vi "Temperature_Analysis.vi"(0 "Temperature_Thresholds":T3, 5 "Boolean":bool) -> (8 "Analysis_Graph":dbl[](graph), 10 "Temperature_Chart":dbl(graph), 15 "Analysis_Data":T2)   [LabVIEW 2020]
doc: "This Vi will act as a temperature analysis VI in which there will be random generation of temperature and then temperature is analysed based on the user inputted threshold input and indicated to the users"
uses:
  Typedefs/Temperature Thresholds.ctl
  Typedefs/AnalysedOutputData.ctl
  Typedefs/Alert_Indicators.ctl
  <vilib>/numeric/Random Number (Range) DBL.vi
panel:
  out "Alert":T1
  in  "error in":errorcluster
  out "error out":errorcluster
  # "Temperature Monitor"
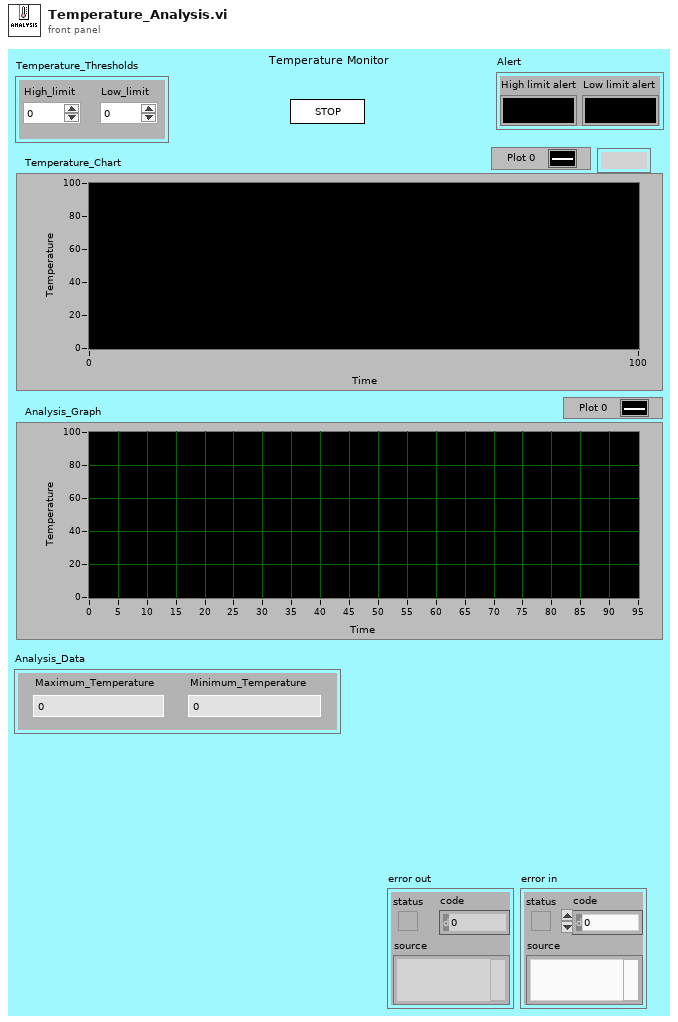
[diagram p1: front panel]
types:
  T1 = typedef "Alert_Indicators.ctl" = cluster{"High limit alert":bool, "Low limit alert":bool}
  T2 = typedef "AnalysedOutputData.ctl" = cluster{"Maximum_Temperature":dbl, "Minimum_Temperature":dbl}
  T3 = typedef "Temperature Thresholds.ctl" = cluster{"High_limit":dbl, "Low_limit":dbl}
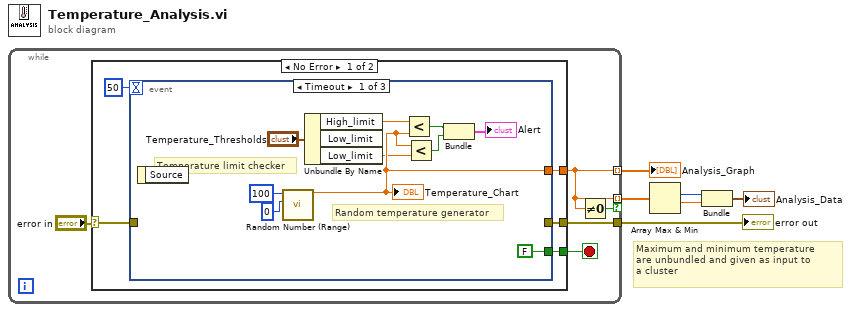
[diagram p0: block diagram]
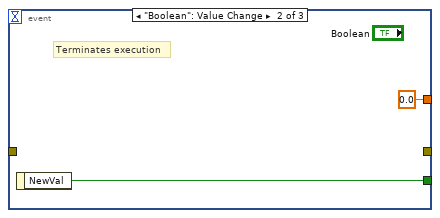
[diagram p2: hidden frame]
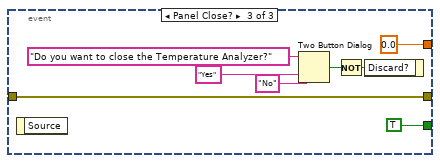
[diagram p3: hidden frame]
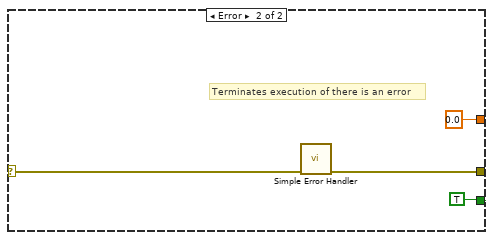
[diagram p4: hidden frame]
diagram:
  # "Maximum and minimum temperature \nare unbundled and given as input to \na cluster"
  n1 = while {
    tunnel: [w7] -> w6 mode=indexing if=w8
    tunnel: [w7] -> w2 mode=indexing
    tunnel: [w10] -> w1
    stop <- w11 stop-if-true
    n2 = case shown="No Error" "error in" {
      selector: "error in" -> [w12 w40]
      tunnel: [w16 0.0 ("number")] -> w7
      tunnel: [w15 TRUE ("NewVal")] -> w11
      tunnel: [w13 w39] -> w10
      frame No Error {
        n3 = event shown="[0] Timeout" {
          selector: _ -> [_ _ _]
          dyn-events: _ -> [_ _ _]
          timeout: 50 -> [_ _ _]
          tunnel: [w26 0.0 ("number") 0.0 ("number")] -> w16
          tunnel: [FALSE ("NewVal") w28 TRUE ("NewVal")] -> w15
          tunnel: [_ _ w29] -> w13
          tunnel: w12 -> [_ _ w29]
          event Timeout {
            # "Temperature limit checker"
            # "Random temperature generator"
            n4 = event-data() -> ()  [unwired: 1 in, 1 out]
            n5 = call-poly <vilib>:"Random Number (Range).vi"("lower bound (0)"=u64 0, "upper bound (100)"=u64 100) -> ("number"=w26:dbl)  [unwired: 9 in]
            "Temperature_Chart" <- w26
            n6 = Unbundle By Name("Temperature_Thresholds") -> ("High_limit"=w24:dbl, "Low_limit"=w23:dbl)  [unwired: 1 out]
            n7 = Less?(x=w24, y=w26) -> (x < y?=w19:bool)
            n8 = Less?(x=w26, y=w23) -> (x < y?=w18:bool)
            n9 = Bundle(w19, w18) -> (→"Alert":cluster{bool, bool})  [unwired: 1 in]
          }
          event "Boolean": Value Change {
            # "Terminates execution"
            n10 = event-data() -> ("NewVal"=w28:bool)  [unwired: 1 in]
          }
          event Panel Close? {
            n11 = event-data() -> ()  [unwired: 1 in, 1 out]
            n12 = Two Button Dialog(message="Do you want to close the Temperature Analyzer?", 1:"No" ("F button name (\"Cancel\")"), 2:"Yes" ("T button name (\"OK\")")) -> (T button?=w31:bool)
            n13 = Not(x=w31) -> (.not. x?=w30:bool)
            n14 = event-data("Discard?"=w30) -> ()  [unwired: 1 in, 1 out]
          }
        }
      }
      frame Error {
        # "Terminates execution of there is an error"
        n15 = call <vilib>:"Simple Error Handler.vi"("error in (no error)"=w40) -> ("error out"=w39:errorcluster)  [unwired: 4 in, 4 out]
      }
    }
    n16 = Not Equal To 0?(x=w7) -> (x != 0?=w8:bool)
  }
  "Analysis_Graph" <- w2
  "error out" <- w1
  n17 = Array Max & Min(array=w6) -> (max index (indices)=w5:i32, min value=w4:dbl)  [unwired: 2 out]
  n18 = Bundle(w5, w4) -> (→"Analysis_Data":cluster{i32, dbl})  [unwired: 1 in]
